vi "Convert_I32toDBL.vi"(9 "Acqu.Indicator":T1={"TrigDelay"=0.0, "Offset"=0, "Resolution"=-32768, "Range (mV)"=0, "Sample Rate"=100000000.0, "Depth"=16384.0, "Segments"=1} {"Segments" min=1 max=1024 step=1; "Sample Rate" format="%.0p"}, 10 "Interger Signal":i32[](array[numeric])) -> (2 "Data in Volts":dbl[](array[numeric]) format="%.2f")   [LabVIEW 2013]
uses:
  ProcessMethods/SignalAverager/DAQParams.ctl
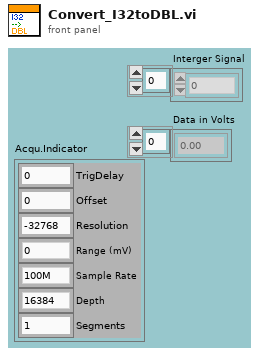
[diagram p1: front panel]
types:
  T1 = typedef "DAQParams.ctl" = cluster{"TrigDelay":dbl, "Offset":i32, "Resolution":i32, "Range (mV)":u32, "Sample Rate":dbl, "Depth":dbl, "Segments":u32}
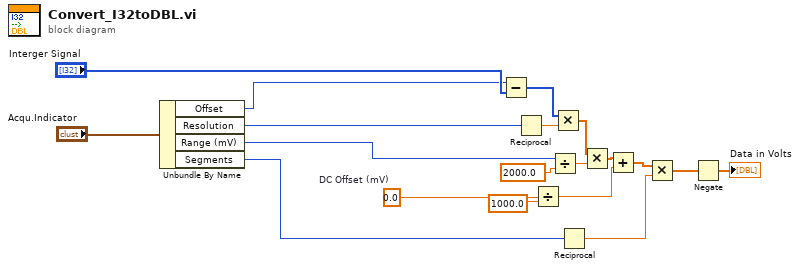
[diagram p0: block diagram]
diagram:
  w2 = 0.0  # DC Offset (mV)
  n1 = Unbundle By Name("Acqu.Indicator") -> ("Offset"=w3:i32, "Resolution"=w4:i32, "Range (mV)"=w5:u32, "Segments"=w1:u32)
  n2 = Subtract(x=w3, y="Interger Signal") -> (x-y=w19:i32[])
  n3 = Reciprocal(x=w4) -> (1/x=w10:dbl)
  n4 = Divide(x=w2, y=1000.0) -> (x/y=w13:dbl)
  n5 = Divide(x=w5, y=2000.0) -> (x/y=w14:dbl)
  n6 = Multiply(x=w19, y=w10) -> (x*y=w15:dbl[])
  n7 = Reciprocal(x=w1) -> (1/x=w8:dbl)
  n8 = Multiply(x=w15, y=w14) -> (x*y=w17:dbl[])
  n9 = Add(x=w17, y=w13) -> (x+y=w12:dbl[])
  n10 = Multiply(x=w12, y=w8) -> (x*y=w9:dbl[])
  n11 = Negate(x=w9) -> (-x=→"Data in Volts":dbl[])
